vi "Initialize_Base64_URL_Encoding.vi"() -> (3 "Base64 URL Encoding":refnum<class "Serializer.Base64.lvclass">)   [LabVIEW 2013, in "Serializer.Base64.lvclass"]
uses:
  Serializer.Base64.lvclass
  Serializer.Base64.lvclass/Serializer.Base64.ctl
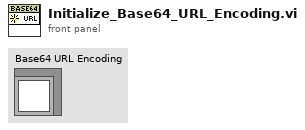
[diagram p1: front panel]
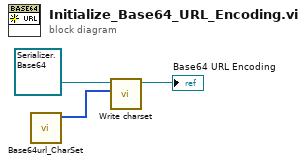
[diagram p0: block diagram]
diagram:
  n1 = call "Base64url_CharSet.vi"() -> ("base64 URL charset"=w2:u8[])  [unwired: 11 in]
  n2 = call "Write charset.vi"("charset"=w2, "Serializer.Base64 in"=refnum<class "Serializer.Base64.lvclass"> refnum ("Serializer.Base64.lvclass")) -> ("Serializer.Base64 out"=→"Base64 URL Encoding":refnum<class "Serializer.Base64.lvclass">)  [unwired: 8 in, 1 out]
